vi "PV Set Pressure Data.vi"(1 "Pressure (mbar)\n0 ==> ur (<1,0e-4mbar)\n1 - 2050 mbar":i16 min=0 max=2050 step=1) -> (0 "Output":string)   [LabVIEW 2024, in "Pfeiffer Vacuum.lvlib"]
uses:
  <instrlib>/Pfeiffer Vacuum/Pfeiffer Vacuum.lvlib
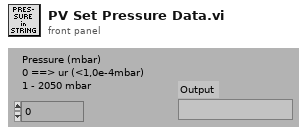
[diagram p1: front panel]
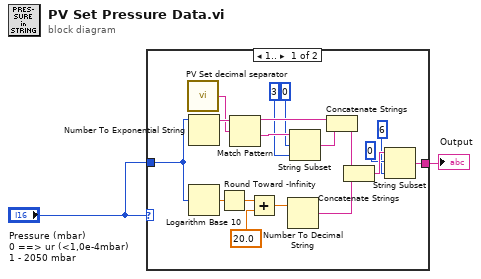
[diagram p0: block diagram]
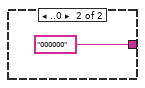
[diagram p2: hidden frame]
diagram:
  n1 = case shown="1.." "Pressure (mbar)\n0 ==> ur (<1,0e-4mbar)\n1 - 2050 mbar" {
    tunnel: [w8 "000000"] -> w2
    tunnel: "Pressure (mbar)\n0 ==> ur (<1,0e-4mbar)\n1 - 2050 mbar" -> [w4 _]
    frame 1.. {
      n2 = call <instrlib>:"PV Set decimal separator.vi"() -> ("decimal separator"=w3:string)
      n3 = Number To Exponential String(number=w4) -> (E-format string=w17:string)  [unwired: 3 in]
      n4 = Logarithm Base 10(1:w4) -> (0:w20:dbl)
      n5 = Round Toward -Infinity(1:w20) -> (0:w19:dbl)
      n6 = Match Pattern(string=w17, regular expression=w3) -> (before substring=w18:string, after substring=w16:string)  [unwired: 1 in, 2 out]
      n7 = Add(x=w19, y=20.0) -> (x+y=w12:dbl)
      n8 = Number To Decimal String(number=w12) -> (decimal integer string=w9:string)  [unwired: 1 in]
      n9 = String Subset(string=w16, offset (0)=0 ("Offset (0)"), length (rest)=3 ("Länge")) -> (substring=w13:string)
      n10 = Concatenate Strings(w18, w13) -> (w10:string)
      n11 = Concatenate Strings(w10, w9) -> (w7:string)
      n12 = String Subset(string=w7, offset (0)=0 ("Offset (0)"), length (rest)=6 ("Länge")) -> (substring=w8:string)
    }
    frame ..0 {
    }
  }
  "Output" <- w2
